vi "Get Target File Folder.vi"(8 "error in (no error)":errorcluster, 11 "ImageLoad in":refnum<class "ImageLoad.lvclass">) -> (0 "error out":errorcluster, 2 "Target File Folder":path, 3 "ImageLoad out":refnum<class "ImageLoad.lvclass">)   [LabVIEW 2015, in "ImageLoad.lvclass"]
uses:
  ImageLoad.lvclass
  ImageLoad.lvclass/ImageLoad.ctl
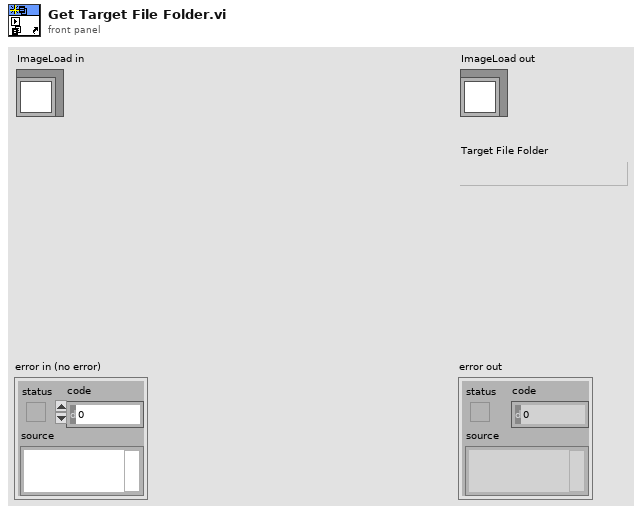
[diagram p1: front panel]
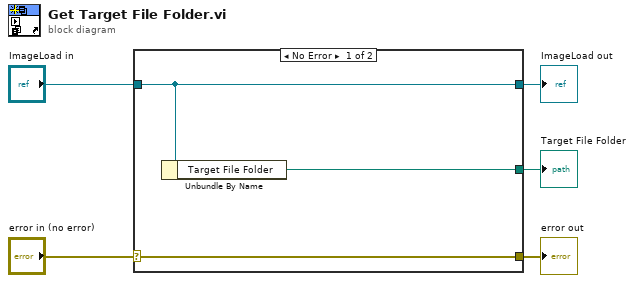
[diagram p0: block diagram]
diagram:
  n1 = case shown="No Error" "error in (no error)" {
    selector: "error in (no error)" -> [w8 w9]
    tunnel: [w8 w9] -> w4
    tunnel: [w7 w10] -> w2
    tunnel: "ImageLoad in" -> [w7 w10]
    tunnel: [w6 _] -> w1
    frame No Error {
      n2 = Unbundle By Name(w7) -> ("Target File Folder"=w6:path)
    }
    frame Error {
    }
  }
  "error out" <- w4
  "ImageLoad out" <- w2
  "Target File Folder" <- w1
